vi "Get Environment.vi"(8 "error in":errorcluster, 11 "Paths":T1) -> (0 "error out":errorcluster, 3 "Environment out":refnum<k24>)   [LabVIEW 2020, in "WebView2 Control.xctl"]
uses:
  WebView2 Control.xctl
  Paths.ctl
  E:/Labview/LV 2020/Libs/LV-WebView2/microsoft.web.webview2/lib/net45/Microsoft.Web.WebView2.Core.dll
  microsoft.web.webview2/lib/net45/Microsoft.Web.WebView2.Core.dll
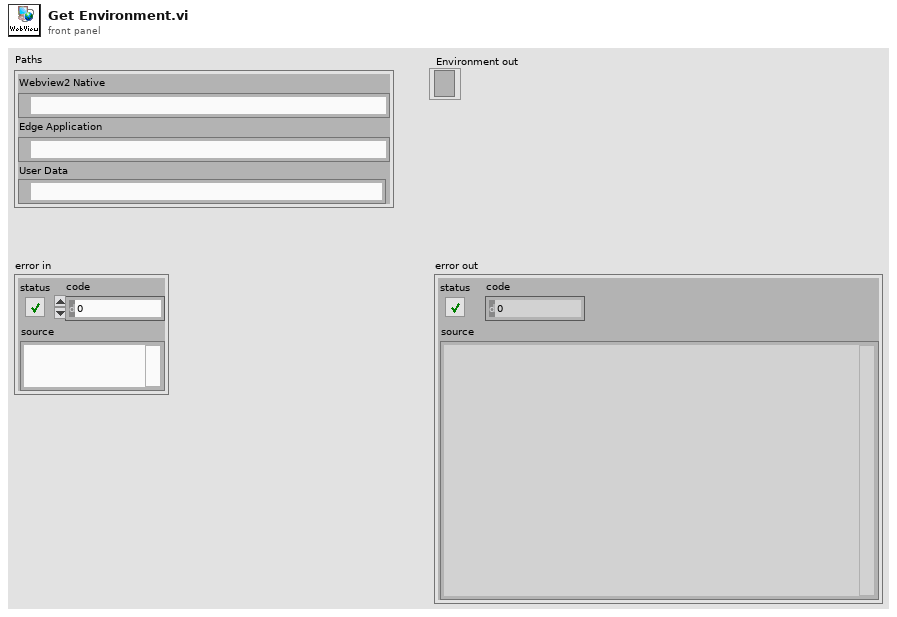
[diagram p1: front panel]
types:
  T1 = typedef "WebView2 Control.xctl/Paths.ctl" = cluster{"Webview2 Native":path, "Edge Application":path, "User Data":path}
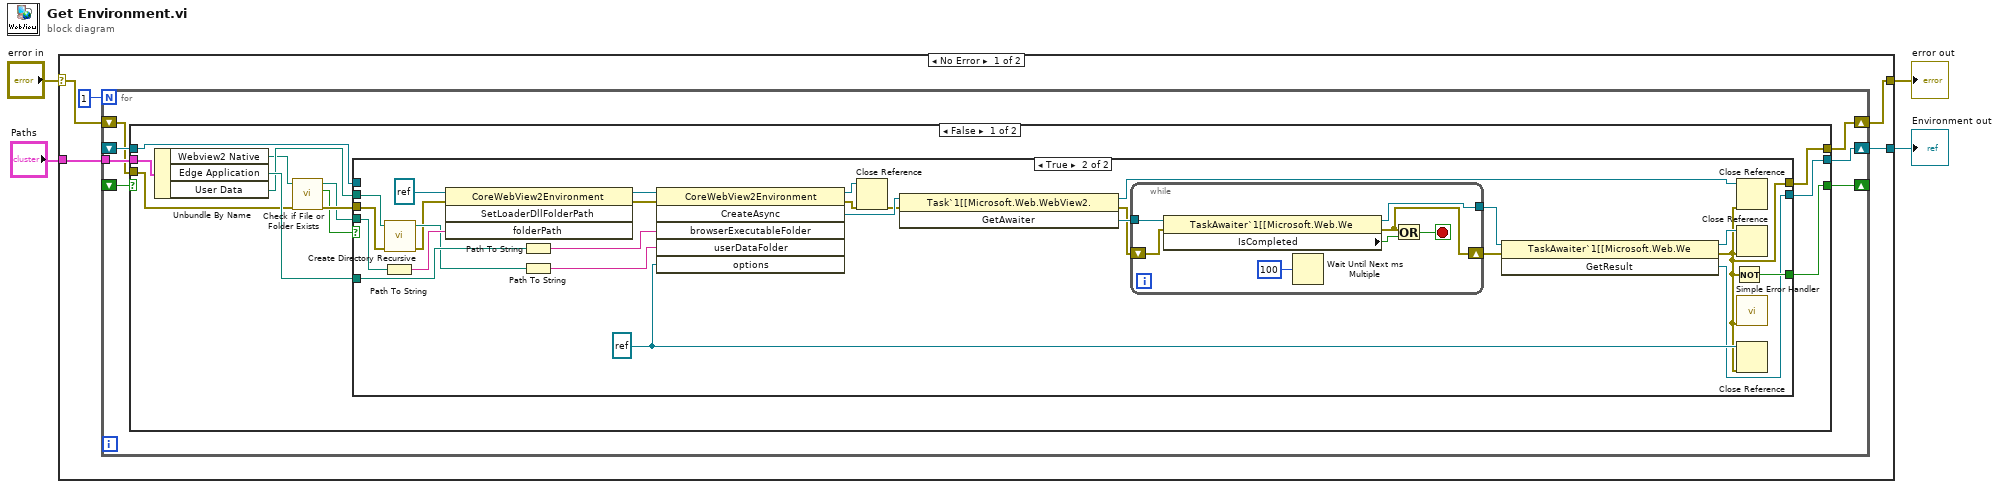
[diagram p0: block diagram]
diagram:
  n1 = case shown="No Error" "error in" {
    selector: "error in" -> [w6 w67]
    tunnel: [w9 w67] -> w4
    tunnel: [w8 _] -> w3
    tunnel: "Paths" -> [w7 _]
    frame No Error {
      n2 = for {
        N: 1 -> [_]
        tunnel: w7 -> [w16]
        shift-right: [w14] -> w8
        shift-left: _ -> [w13]
        shift-right: [w15] -> w9
        shift-left: w6 -> [w12]
        shift-right: [w11] -> _
        shift-left: _ -> [w10]
        n3 = case shown="False" w10 {
          selector: w10 -> [_ w64]
          tunnel: w16 -> [w26 _]
          tunnel: [w23 w65] -> w15
          tunnel: [w25 w66] -> w14
          tunnel: w13 -> [w17 w66]
          tunnel: w12 -> [w24 w65]
          tunnel: [w22 w64] -> w11
          frame False {
            n4 = Unbundle By Name(w26) -> ("Webview2 Native"=w20:path, "Edge Application"=w28:path, "User Data"=w27:path)
            n5 = call <vilib>:"Check if File or Folder Exists.vi"("error in (no error)"=w24, "path"=w20) -> ("error out"=w21:errorcluster, "file or folder exists?"=w18:bool, "dup path"=w19:path)  [unwired: 7 in]
            n6 = case shown="True" w18 {
              tunnel: w28 -> [_ w50]
              tunnel: w27 -> [_ w41]
              tunnel: [w30 w35] -> w25
              tunnel: [w29 w31] -> w23
              tunnel: [_ w44] -> w22
              tunnel: w21 -> [w29 w42]
              tunnel: w19 -> [_ w43]
              tunnel: w17 -> [w30 _]
              frame False {
              }
              frame True {
                w38 = refnum<k24> refnum ("options")
                n7 = Path To String(path=w43) -> (string=w53:string)
                n8 = call <vilib>:"Create Directory Recursive.vi"("error in (no error)"=w42, "directory"=w41) -> ("error out"=w39:errorcluster, "directory copy"=w40:path)  [unwired: 3 in, 1 out]
                n9 = invoke class="CoreWebView2Environment" method="SetLoaderDllFolderPath"(reference=refnum<k24> refnum ("environment"), error in=w39, "folderPath"=w53) -> (reference out=w55:refnum<k24>, error out=w54:errorcluster)  [unwired: 1 in, 2 out]
                n10 = Path To String(path=w50) -> (string=w52:string)
                n11 = Path To String(path=w40) -> (string=w37:string)
                n12 = invoke class="CoreWebView2Environment" method="CreateAsync"(reference=w55, error in=w54, "browserExecutableFolder"=w52, "userDataFolder"=w37, "options"=w38) -> (reference out=w33:refnum<k24>, error out=w46:errorcluster, "CreateAsync"=w51:refnum<k24>)  [unwired: 1 in, 3 out]
                n13 = Close Reference(reference=w33, error in (no error)=w46) -> (error out=w34:errorcluster)
                n14 = invoke class="Task`1[[Microsoft.Web.WebView2." method="GetAwaiter"(reference=w51, error in=w34) -> (reference out=w45:refnum<k24>, error out=w48:errorcluster, "GetAwaiter"=w49:refnum<k24>)  [unwired: 1 in]
                n15 = while {
                  tunnel: w49 -> [w62]
                  shift-right: [w57] -> w32
                  shift-left: w48 -> [w63]
                  tunnel: [w59] -> w47
                  stop <- w58 stop-if-true
                  n16 = property class="TaskAwaiter`1[[Microsoft.Web.We"(reference=w62, error in=w63) -> (reference out=w59:refnum<k24>, error out=w57:errorcluster, "IsCompleted"=w60:bool)
                  n17 = Wait Until Next ms Multiple(millisecond multiple=u32 100) -> ()  [unwired: 1 out]
                  n18 = Or(x=w57, y=w60) -> (x .or. y?=w58:bool)
                }
                n19 = invoke class="TaskAwaiter`1[[Microsoft.Web.We" method="GetResult"(reference=w47, error in=w32) -> (reference out=w36:refnum<k24>, error out=w31:errorcluster, "GetResult"=w35:refnum<k24>)  [unwired: 1 in]
                n20 = Not(x=w31) -> (.not. x?=w44:bool)
                n21 = Close Reference(reference=w45, error in (no error)=w31) -> ()  [unwired: 1 out]
                n22 = Close Reference(reference=w36, error in (no error)=w31) -> ()  [unwired: 1 out]
                n23 = call <vilib>:"Simple Error Handler.vi"("error in (no error)"=w31) -> ()  [unwired: 4 in, 5 out]
                n24 = Close Reference(reference=w38, error in (no error)=w31) -> ()  [unwired: 1 out]
              }
            }
          }
          frame True {
          }
        }
      }
    }
    frame Error {
    }
  }
  "error out" <- w4
  "Environment out" <- w3
